vi "MultiStatus.vi"(0 "VisaCluster":T1, 11 "error in (no error)":errorcluster) -> (4 "VisaCluster":T1, 8 "Answer":string, 10 "Multi":bool, 15 "error out":errorcluster)   [LabVIEW 2014, in "FH 55.lvlib"]
uses:
  FH 55.lvlib
  TypeDef/VisaCluster.ctl
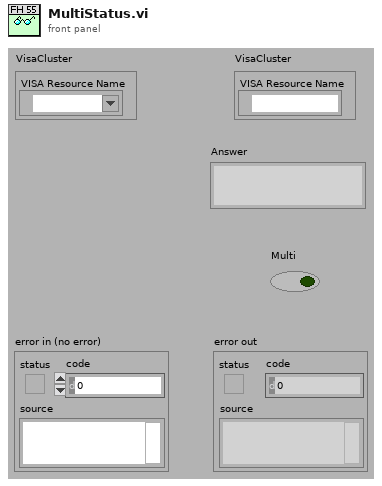
[diagram p1: front panel]
types:
  T1 = typedef "FH 55.lvlib/VisaCluster.ctl" = cluster{"VISA Resource Name":refnum<visa-resource-name>}
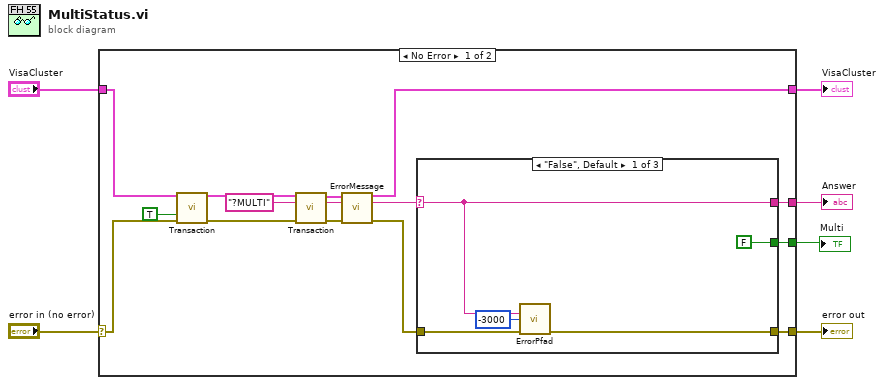
[diagram p0: block diagram]
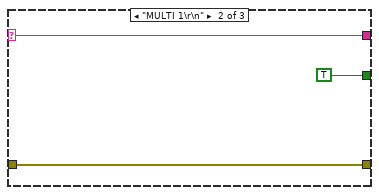
[diagram p2: hidden frame]
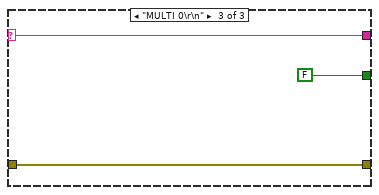
[diagram p3: hidden frame]
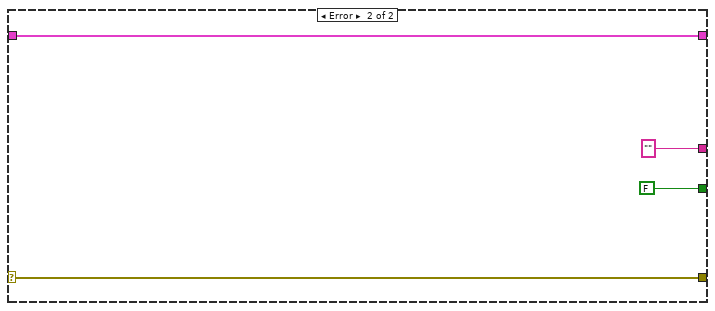
[diagram p4: hidden frame]
diagram:
  n1 = case shown="No Error" "error in (no error)" {
    selector: "error in (no error)" -> [w17 w35]
    tunnel: "VisaCluster" -> [w15 w36]
    tunnel: [w21 w36] -> w2
    tunnel: [w10 w35] -> w4
    tunnel: [w9 ""] -> w3
    tunnel: [w12 FALSE] -> w1
    frame No Error {
      n2 = call "Transaction.vi"("VisaCluster"=w15, "Read Only? (False)"=TRUE, "error in (no error)"=w17) -> ("VisaCluster"=w14:T1, "error out"=w16:errorcluster)  [unwired: 9 in, 2 out]
      n3 = call "Transaction.vi"("VisaCluster"=w14, "Command"="?MULTI", "error in (no error)"=w16) -> ("VisaCluster"=w19:T1, "Answer"=w7:string, "error out"=w20:errorcluster)  [unwired: 9 in, 1 out]
      n4 = call "ErrorMessage.vi"("VisaCluster"=w19, "Message In"=w7, "error in (no error)"=w20) -> ("VisaCluster"=w21:T1, "Message Out"=w8:string, "error out"=w11:errorcluster)  [unwired: 10 in]
      n5 = case shown="\"False\", Default" w8 {
        selector: w8 -> [w22 w27 w31]
        tunnel: [FALSE TRUE FALSE] -> w12
        tunnel: w11 -> [w25 w28 w30]
        tunnel: [w24 w28 w30] -> w10
        tunnel: [w22 w27 w31] -> w9
        frame "False", Default {
          n6 = call "ErrorPfad.vi"("Message In"=w22, "Numeric"=-3000, "error in (no error)"=w25) -> ("error out"=w24:errorcluster)  [unwired: 11 in, 1 out]
        }
        frame "MULTI 1\r\n" {
        }
        frame "MULTI 0\r\n" {
        }
      }
    }
    frame Error {
    }
  }
  "error out" <- w4
  "Answer" <- w3
  "VisaCluster" <- w2
  "Multi" <- w1
